vi "MC600Demo.vi"(0 "ComPort":i16, 1 "axis":i16, 2 "AccSpeed":sgl, 3 "AxisStyle":i16, 4 "InitSpeed":sgl, 5 "Speed":sgl, 6 "dir":i16, 7 "step":sgl, 8 "workstate":i16, 9 "StepAngle":sgl, 10 "x":sgl, 12 "state":i16) -> (14 "字符串":string="打开失败")   [LabVIEW 2015]
panel:
  in  "ZOLIXMC6002":refnum<k7>(container)
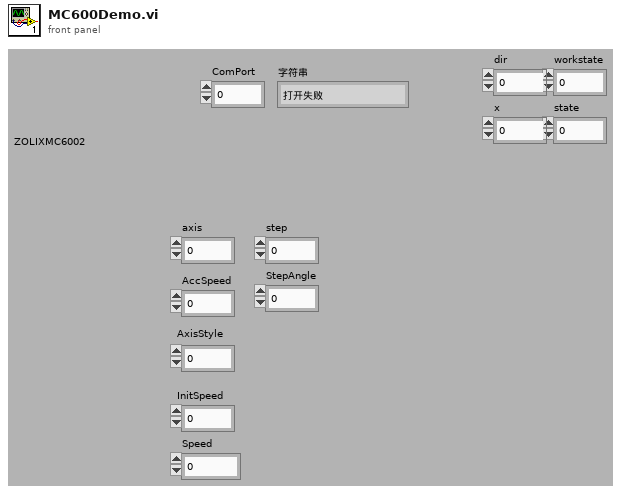
[diagram p1: front panel]
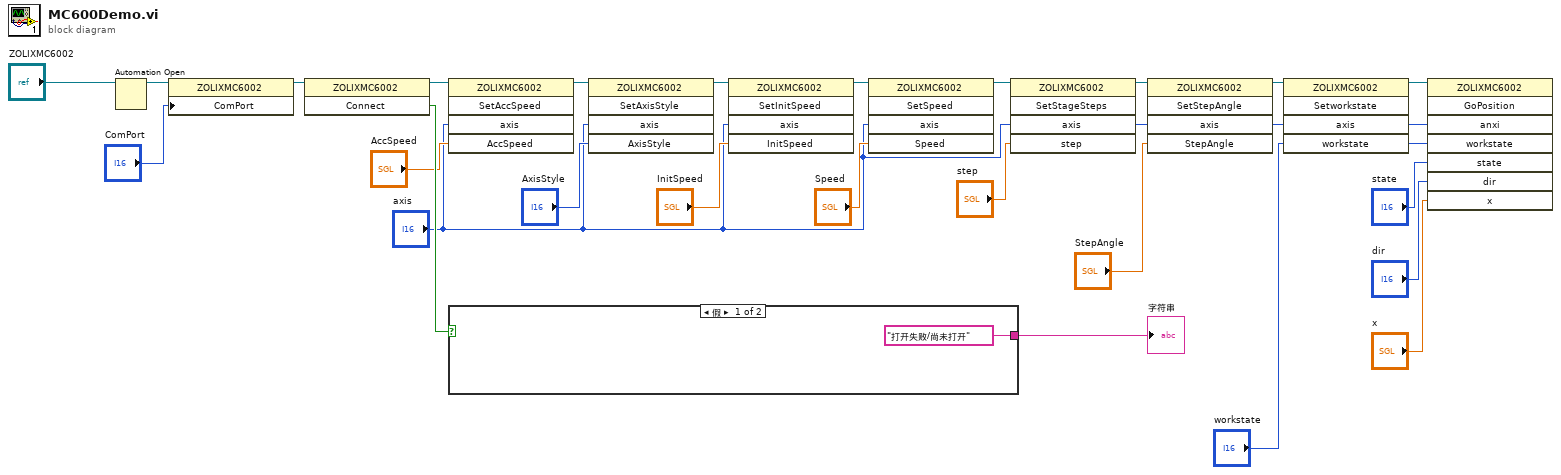
[diagram p0: block diagram]
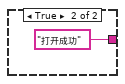
[diagram p2: hidden frame]
diagram:
  n1 = Automation Open(Automation Refnum="ZOLIXMC6002") -> (Automation Refnum=w28:refnum<k7>)  [unwired: 3 in, 1 out]
  n2 = property class="ZOLIXMC6002"(reference=w28, "ComPort"="ComPort") -> (reference out=w26:refnum<k7>)  [unwired: 1 in, 1 out]
  n3 = invoke class="ZOLIXMC6002" method="Connect"(reference=w26) -> (reference out=w2:refnum<k7>, "Connect"=w25:bool)  [unwired: 2 in, 1 out]
  n4 = invoke class="ZOLIXMC6002" method="SetAccSpeed"(reference=w2, "axis"="axis", "AccSpeed"="AccSpeed") -> (reference out=w22:refnum<k7>)  [unwired: 2 in, 4 out]
  n5 = case shown="假" w25 {
    tunnel: ["打开失败/尚未打开" "打开成功"] -> w24
    frame False {
    }
    frame True {
    }
  }
  "字符串" <- w24
  n6 = invoke class="ZOLIXMC6002" method="SetAxisStyle"(reference=w22, "axis"="axis", "AxisStyle"="AxisStyle") -> (reference out=w20:refnum<k7>)  [unwired: 2 in, 4 out]
  n7 = invoke class="ZOLIXMC6002" method="SetInitSpeed"(reference=w20, "axis"="axis", "InitSpeed"="InitSpeed") -> (reference out=w18:refnum<k7>)  [unwired: 2 in, 4 out]
  n8 = invoke class="ZOLIXMC6002" method="SetSpeed"(reference=w18, "axis"="axis", "Speed"="Speed") -> (reference out=w16:refnum<k7>)  [unwired: 2 in, 4 out]
  n9 = invoke class="ZOLIXMC6002" method="SetStageSteps"(reference=w16, "axis"="axis", "step"="step") -> (reference out=w14:refnum<k7>, "axis"=w13:i16)  [unwired: 2 in, 3 out]
  n10 = invoke class="ZOLIXMC6002" method="SetStepAngle"(reference=w14, "axis"=w13, "StepAngle"="StepAngle") -> (reference out=w11:refnum<k7>, "axis"=w10:i16)  [unwired: 2 in, 3 out]
  n11 = invoke class="ZOLIXMC6002" method="Setworkstate"(reference=w11, "axis"=w10, "workstate"="workstate") -> (reference out=w8:refnum<k7>, "axis"=w7:i16, "workstate"=w6:i16)  [unwired: 2 in, 2 out]
  n12 = invoke class="ZOLIXMC6002" method="GoPosition"(reference=w8, "anxi"=w7, "workstate"=w6, "state"="state", "dir"="dir", "x"="x") -> ()  [unwired: 2 in, 8 out]
